vi "Numeric with Units.vi"() -> ()   [LabVIEW 2023]
doc: "This example shows how to configure units on numeric controls and indicators, and use the Unit Label property to programmatically read and write unit label values."
panel:
  out "Far distance":dbl[unit] format="%.2f"
  out "Near distance":dbl[unit] format="%.2f"
  out "Hyperfocal distance":dbl[unit] format="%.2f"
  in  "focus distance":dbl[unit]=6.096
  in  "aperture":dbl=2.8 format="%.1f"
  in  "lens focal length":dbl[unit]=0.05
  # "Overview: Demonstrates how to configure Units on numeric controls and indicators.\nInstructions:\n1. Run the VI. The 'distance' calculations are returned in the same units as specified by the focus distance control.\n2. Double-click the 'ft' unit on the focus distance control and change it to 'm' for meters. Notice that the value in the control changes to match the new unit.\n3. Run the VI again. The 'distance' calculations are now returned in meters because their units are programmatically updated to match the units of the focus distance control."
  # "Changing the units of the focus distance control will result in the units of the 'distance' indicators changing when the VI runs."
  # "Right-click a numeric control or indicator and select Visible Items > Unit Label to show the units."
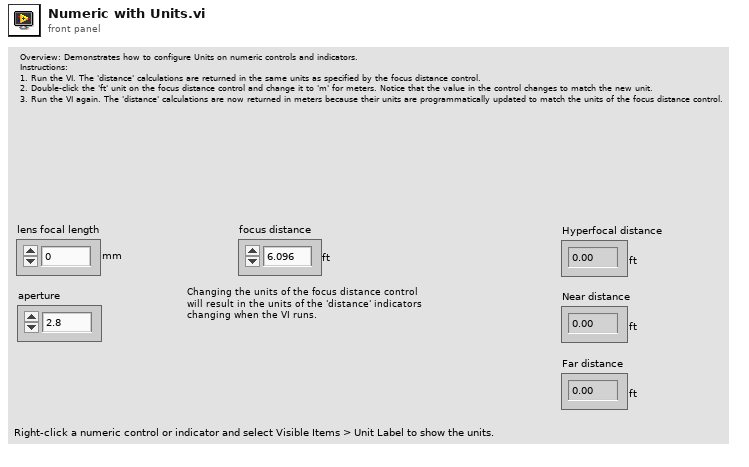
[diagram p1: front panel]
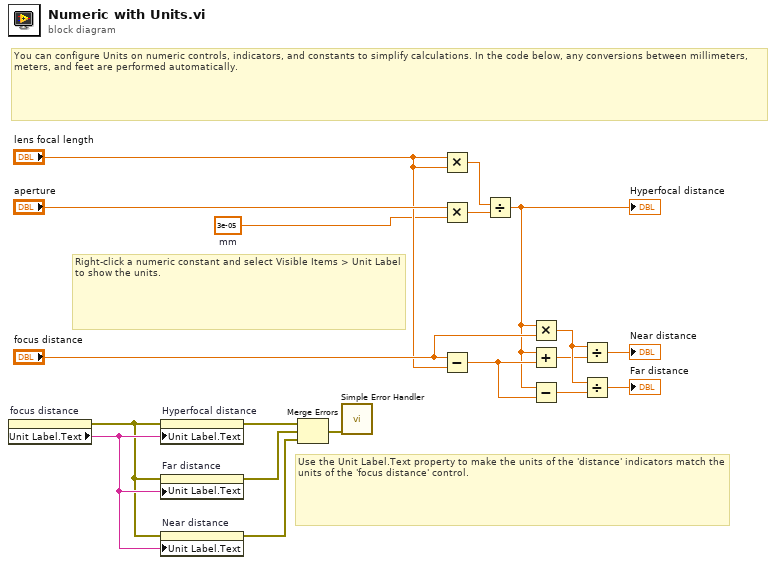
[diagram p0: block diagram]
diagram:
  w1 = dbl[unit] 3e-05  # mm
  # "You can configure Units on numeric controls, indicators, and constants to simplify calculations. In the code below, any conversions between millimeters, meters, and feet are performed automatically."
  # "Use the Unit Label.Text property to make the units of the 'distance' indicators match the units of the 'focus distance' control."
  # "Right-click a numeric constant and select Visible Items > Unit Label to show the units."
  n1 = property on="focus distance" class="Digital (strict)"() -> (error out=w6:errorcluster, "Unit Label.Text"=w7:string)  [unwired: 2 in, 1 out]
  n2 = property on="Hyperfocal distance" class="Digital (strict)"(error in=w6, "Unit Label.Text"=w7) -> (error out=w5:errorcluster)  [unwired: 1 in, 1 out]
  n3 = property on="Far distance" class="Digital (strict)"(error in=w6, "Unit Label.Text"=w7) -> (error out=w3:errorcluster)  [unwired: 1 in, 1 out]
  n4 = property on="Near distance" class="Digital (strict)"(error in=w6, "Unit Label.Text"=w7) -> (error out=w2:errorcluster)  [unwired: 1 in, 1 out]
  n5 = Merge Errors(w5, w3, w2) -> (w4:errorcluster)
  n6 = call <vilib>:"Simple Error Handler.vi"("error in (no error)"=w4) -> ()  [unwired: 4 in, 5 out]
  n7 = Multiply(x="lens focal length", y="lens focal length") -> (x*y=w18:dbl[unit])
  n8 = Multiply(x="aperture", y=w1) -> (x*y=w17:dbl[unit])
  n9 = Subtract(x="focus distance", y="lens focal length") -> (x-y=w14:dbl[unit])
  n10 = Divide(x=w18, y=w17) -> (x/y=w8:dbl[unit])
  "Hyperfocal distance" <- w8
  n11 = Multiply(x=w8, y="focus distance") -> (x*y=w13:dbl[unit])
  n12 = Add(x=w8, y=w14) -> (x+y=w12:dbl[unit])
  n13 = Subtract(x=w8, y=w14) -> (x-y=w11:dbl[unit])
  n14 = Divide(x=w13, y=w12) -> (x/y=→"Near distance":dbl[unit])
  n15 = Divide(x=w13, y=w11) -> (x/y=→"Far distance":dbl[unit])
